vi "Get Execution Unit Inline.vi"(8 "error in":errorcluster, 11 "custom device ref":T1 format="%.0x") -> (0 "error out":errorcluster, 1 "Inline Rx Execution":bool caption="Inline Rx Monitor  Execution", 2 "Inline Tx Generic":bool caption="Inline Tx Generic Execution", 3 "custom device ref out":T1 format="%.0x", 5 "Inline Rx UDP":bool caption="Inline Rx UDP Execution", 7 "Inline Tx UDP":bool caption="Inline Tx UDP Execution")   [LabVIEW 2020, in "AIM ARINC 664 Scripting.lvlib"]
uses:
  AIM ARINC 664 Scripting.lvlib
  <vilib>/NI VeriStand/Custom Device API/Custom Device Item Ref.ctl
  Constants.vi
  <vilib>/NI VeriStand/Custom Device API/Get Item Property (Boolean).vi
  <vilib>/NI VeriStand/Custom Device API/Custom Device API.lvlib
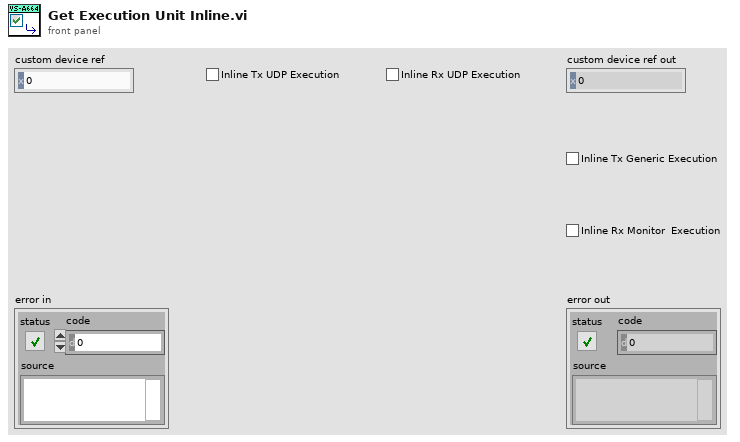
[diagram p1: front panel]
types:
  T1 = typedef "Custom Device API.lvlib/Custom Device Item Ref.ctl" = u64
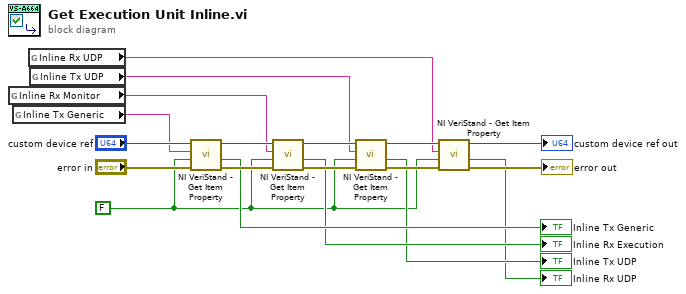
[diagram p0: block diagram]
diagram:
  w1 = FALSE ("Default Value")
  n1 = global read "Constants.vi" "Inline Rx Monitor"() -> (w8:string)
  n2 = global read "Constants.vi" "Inline Tx Generic"() -> (w9:string)
  n3 = global read "Constants.vi" "Inline Rx UDP"() -> (w6:string)
  n4 = global read "Constants.vi" "Inline Tx UDP"() -> (w7:string)
  n5 = call-poly <vilib>:"NI VeriStand - Get Item Property.vi"("error in (no error)"="error in", "Default Value"=w1, "Property Name"=w9, "Item Ref in"="custom device ref") -> ("error out"=w13:errorcluster, "Value"=→"Inline Tx Generic":bool, "Item Ref out"=w18:T1)  [unwired: 4 in, 1 out]
  n6 = call-poly <vilib>:"NI VeriStand - Get Item Property.vi"("error in (no error)"=w13, "Default Value"=w1, "Property Name"=w8, "Item Ref in"=w18) -> ("error out"=w12:errorcluster, "Value"=→"Inline Rx Execution":bool, "Item Ref out"=w17:T1)  [unwired: 4 in, 1 out]
  n7 = call-poly <vilib>:"NI VeriStand - Get Item Property.vi"("error in (no error)"=w12, "Default Value"=w1, "Property Name"=w7, "Item Ref in"=w17) -> ("error out"=w11:errorcluster, "Value"=→"Inline Tx UDP":bool, "Item Ref out"=w16:T1)  [unwired: 4 in, 1 out]
  n8 = call-poly <vilib>:"NI VeriStand - Get Item Property.vi"("error in (no error)"=w11, "Default Value"=w1, "Property Name"=w6, "Item Ref in"=w16) -> ("error out"=→"error out":errorcluster, "Value"=→"Inline Rx UDP":bool, "Item Ref out"=→"custom device ref out":T1)  [unwired: 4 in, 1 out]
